vi "Proceed connection state.vi"(8 "error in (no error)":errorcluster, 10 "Proxy.lvlib:Proxy Status Msg.lvclass":refnum<class "Proxy Status Msg.lvclass">, 11 "Alice in":refnum<class "Alice.lvclass">) -> (0 "error out":errorcluster, 3 "Alice out":refnum<class "Alice.lvclass">)   [LabVIEW 2014, in "Alice.lvlib" / "Alice.lvclass"]
uses:
  Alice.lvclass
  Proxy/Proxy Messages/Proxy Status Msg/Proxy Status Msg.lvclass
  Proxy/Proxy Messages/Proxy Status Msg/Proxy Status Msg.lvclass/Proxy Status Msg.ctl
panel:
  out "Name":string
  out "Writer":bool
  out "Reader":bool
  out "proxy error":errorcluster
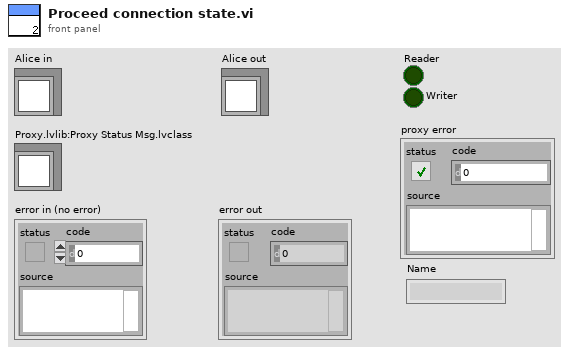
[diagram p1: front panel]
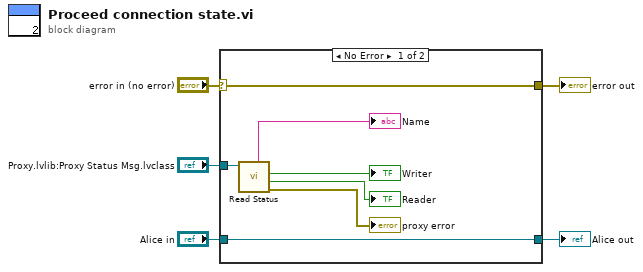
[diagram p0: block diagram]
diagram:
  n1 = case shown="No Error" "error in (no error)" {
    selector: "error in (no error)" -> [w11 w14]
    tunnel: [w11 w14] -> w4
    tunnel: [w12 w13] -> w2
    tunnel: "Alice in" -> [w12 w13]
    tunnel: "Proxy.lvlib:Proxy Status Msg.lvclass" -> [w10 _]
    frame No Error {
      n2 = call "Read Status.vi"("Proxy Status Msg in"=w10) -> ("proxy error"=→"proxy error":errorcluster, "Reader"=→"Reader":bool, "Writer"=→"Writer":bool, "Name"=→"Name":string)  [unwired: 6 in, 1 out]
    }
    frame Error {
    }
  }
  "error out" <- w4
  "Alice out" <- w2
